vi "gfitsio-read-key-double.vi"(7 "keyname":string, 8 "error in (no error)":errorcluster, 9 "default value":dbl, 11 "gfits refnum":T1) -> (0 "error out":errorcluster, 1 "comment":string, 2 "value":dbl, 3 "dup gfits refnum":T1, 4 "units":string)   [LabVIEW 2023, in "gfitsio.lvlib"]
doc: "Return the specified keyword. <B>default value</B> specifies the desired returned data type of the keyword value. Data type conversion will be performed for numeric values if the keyword value does not have the same data type. If the keyword does not exist or an error occurs <B>value</B> will be equal to <B>default value</B>."
uses:
  gfitsio.lvlib
  cfitsio-datatypes.ctl
  gfitsio.dll
  gfitsio-refnum.ctl
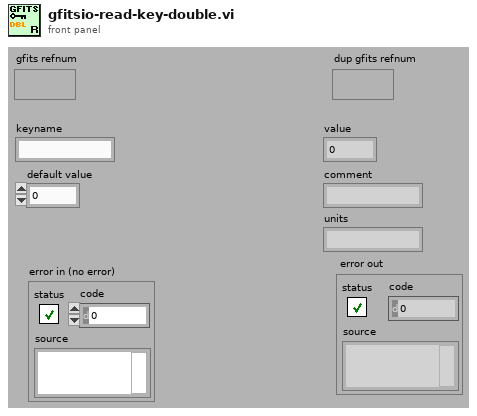
[diagram p1: front panel]
types:
  T1 = typedef "gfitsio.lvlib/gfitsio-refnum.ctl" = refnum<k1>
  T2 = typedef "gfitsio.lvlib/cfitsio-datatypes.ctl" = i32
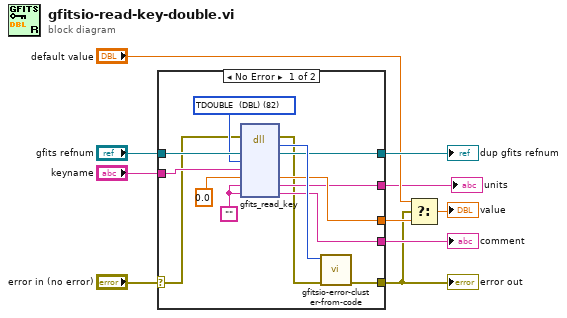
[diagram p0: block diagram]
diagram:
  n1 = case shown="No Error" "error in (no error)" {
    selector: "error in (no error)" -> [w12 w25]
    tunnel: [w22 w25] -> w4
    tunnel: "gfits refnum" -> [w20 w24]
    tunnel: [w21 w24] -> w9
    tunnel: "keyname" -> [w18 _]
    tunnel: [w16 _] -> w5
    tunnel: [w14 _] -> w6
    tunnel: [w15 _] -> w1
    frame No Error {
      w13 = ""
      w19 = T2 82 items=["TBIT"=1, "TBYTE  (U8)"=11, "TSBYTE  (I8)"=12, "TLOGICAL"=14, "TSTRING"=16, "TUSHORT  (U16)"=20, "TSHORT  (I16)"=21, "TUINT"=31, "TULONG  (U32)"=40, "TLONG  (I32)"=41, "TFLOAT  (SGL)"=42, "TLONGLONG  (I64)"=81, "TDOUBLE  (DBL)"=82, "TCOMPLEX  (CSG)"=83, "TDOUBLECOMPLEX  (CDB)"=163] ("cfitsio datatype")
      n2 = dll-call lib="gfitsio.dll" fn="gfits_read_key"(error in=w12, "refnum"=w20, "datatype"=w19, "keyname"=w18, "value"=0.0, "units"=w13, "comment"=w13) -> (error out=w11:errorcluster, w23:i32, "refnum"=w21:T1, "value"=w16:dbl, "units"=w15:string, "comment"=w14:string)  [unwired: 4 in, 1 out]
      n3 = call "gfitsio-error-cluster-from-code.vi"("error in (no error)"=w11, "error code"=w23) -> ("error out"=w22:errorcluster)  [unwired: 9 out]
    }
    frame Error {
    }
  }
  "error out" <- w4
  "dup gfits refnum" <- w9
  "comment" <- w6
  "units" <- w1
  n4 = Select(t="default value", s=w4, f=w5) -> (s? t:f=→"value":dbl)
